vi "Led Comm.vi"() -> ()   [LabVIEW 2019]
uses:
  <vilib>/Rock Robotics/WPI/DriverStation/WPI_DriverStationRobotMode2.ctl
  <vilib>/Rock Robotics/SystemInterfaces/DIO/FPGA_DIOChannel.ctl
  Robot Global Data.vi
panel:
  in  "number":i32
  in  "Time Left":sgl
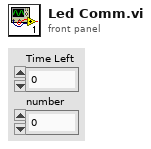
[diagram p1: front panel]
types:
  T1 = typedef "FPGA_DIOChannel.ctl" = enum8{"DIO 0", "DIO 1", "DIO 2", "DIO 3", "DIO 4", "DIO 5", "DIO 6", "DIO 7", "DIO 8", "DIO 9", "DIO MXP 0", "DIO MXP 1", "DIO MXP 2", "DIO MXP 3", "DIO MXP 4", "DIO MXP 5", "DIO MXP 6", "DIO MXP 7", "DIO MXP 8", "DIO MXP 9", "DIO MXP 10", "DIO MXP 11", "DIO MXP 12", "DIO MXP 13", "DIO MXP 14", "DIO MXP 15", "SPI Port CS1", "SPI Port CS2", "SPI Port CS3", "SPI Port MISO", "SPI Port MOSI", "Invalid"}
  T2 = typedef "WPI_DriverStationRobotMode2.ctl" = enum16{"Autonomous Disabled", "Autonomous Enabled", "Teleop Disabled", "Teleop Enabled", "Disconnected", "Finish", "Test Disabled", "Test Enabled", "Emergency Stopped"}
  T3 = typedef "WPI_DigitalOutputDevRef.ctl" = cluster{"DIO Channel":T1, "DevStatus":errorcluster}
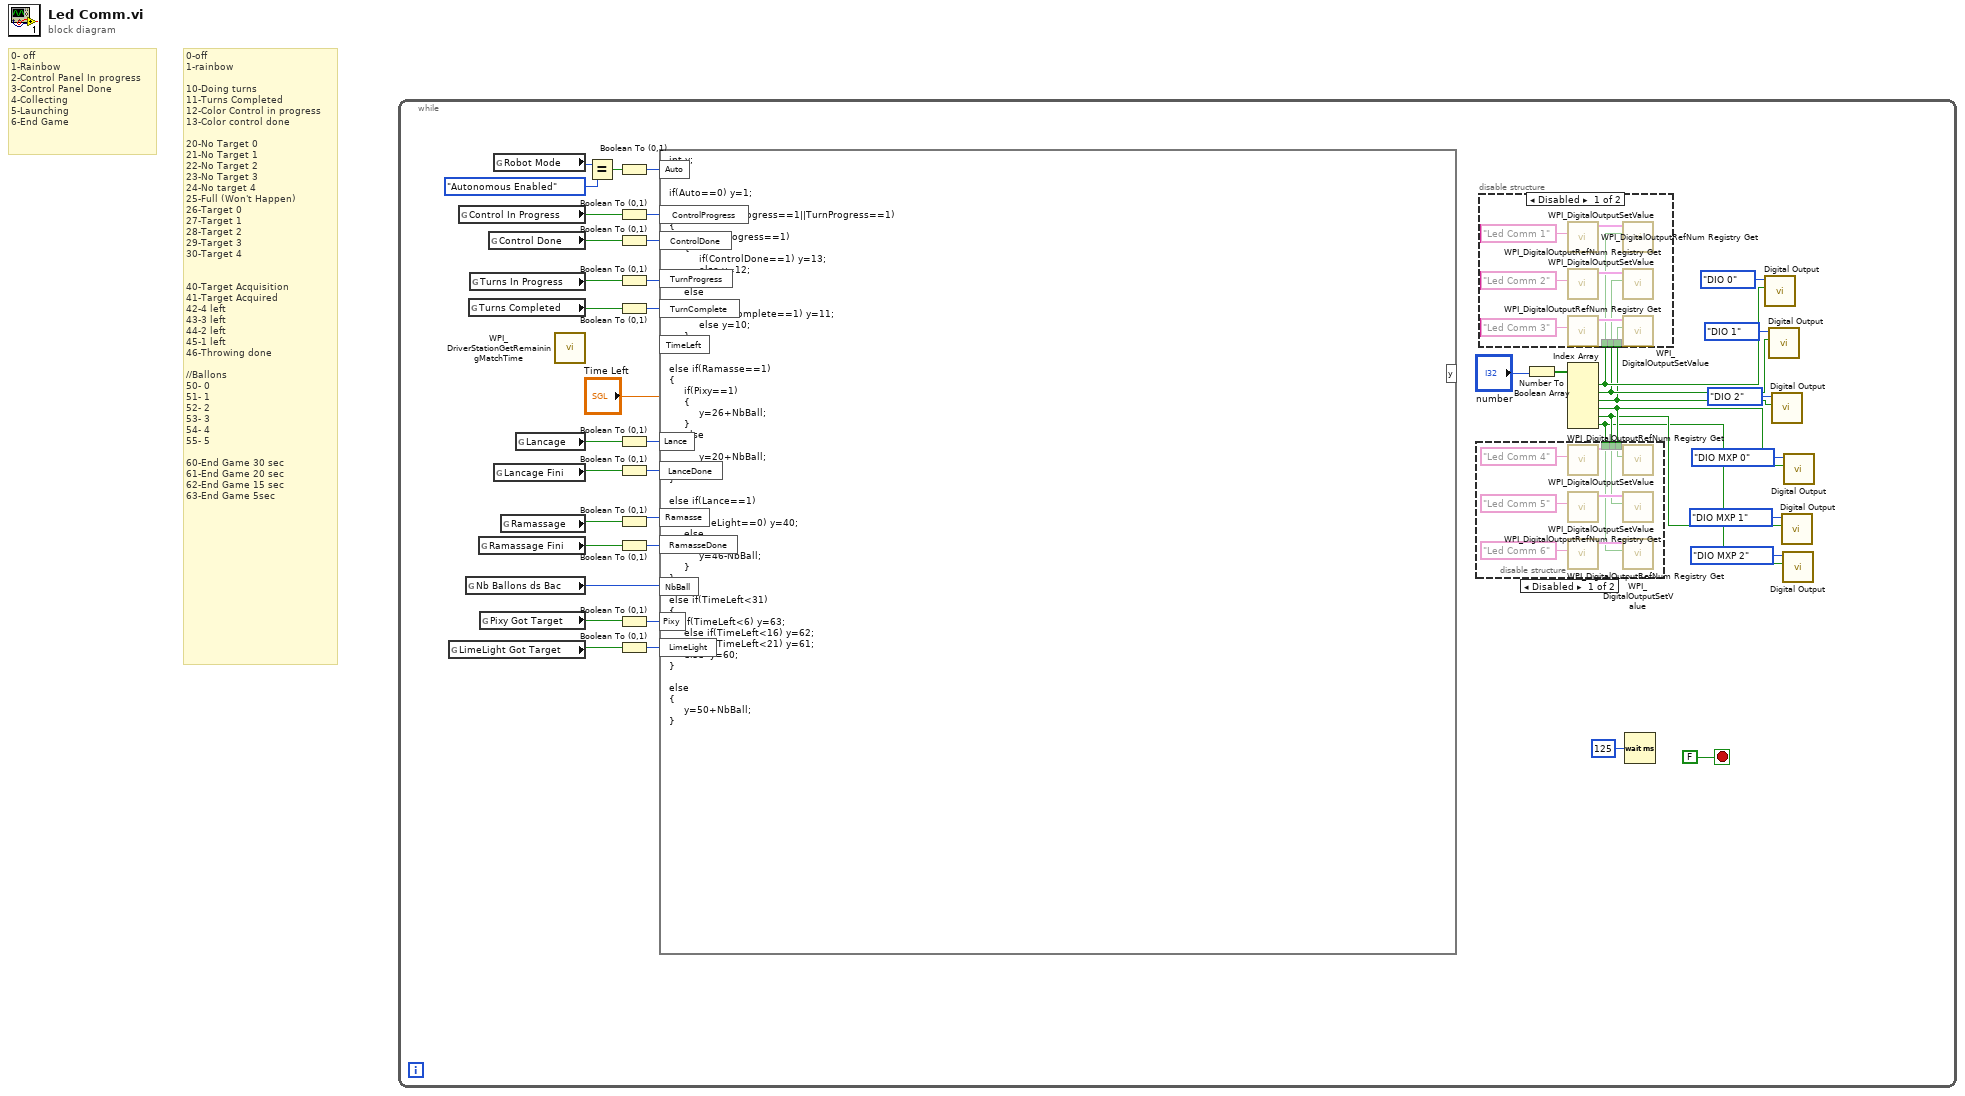
[diagram p0: block diagram]
diagram:
  # "0-off\n1-rainbow\n\n10-Doing turns\n11-Turns Completed\n12-Color Control in progress\n13-Color control done\n\n20-No Target 0\n21-No Target 1\n22-No Target 2\n23-No Target 3\n24-No target 4\n25-Full (Won't Happen)\n26-Target 0\n27-Target 1\n28-Target 2\n29-Target 3\n30-Target 4\n\n\n40-Target Acquisition\n41-Target Acquired\n42-4 left\n43-3 left\n44-2 left\n45-1 left\n46-Throwing done\n\n//Ballons\n50- 0\n51- 1\n52- 2\n53- 3\n54- 4\n55- 5\n\n60-End Game 30 sec\n61-End Game 20 sec\n62-End Game 15 sec\n63-End Game 5sec"
  # "0- off\n1-Rainbow\n2-Control Panel In progress\n3-Control Panel Done\n4-Collecting\n5-Launching\n6-End Game"
  n1 = while {
    stop <- FALSE stop-if-true
    n2 = global read "Robot Global Data.vi" "LimeLight Got Target"() -> (w23:bool)
    n3 = global read "Robot Global Data.vi" "Control In Progress"() -> (w18:bool)
    n4 = global read "Robot Global Data.vi" "Nb Ballons ds Bac"() -> (w24:u8)
    n5 = global read "Robot Global Data.vi" "Turns Completed"() -> (w35:bool)
    n6 = global read "Robot Global Data.vi" "Turns In Progress"() -> (w19:bool)
    n7 = global read "Robot Global Data.vi" "Ramassage Fini"() -> (w34:bool)
    n8 = global read "Robot Global Data.vi" "Pixy Got Target"() -> (w22:bool)
    n9 = global read "Robot Global Data.vi" "Control Done"() -> (w40:bool)
    n10 = global read "Robot Global Data.vi" "Robot Mode"() -> (w38:T2)
    n11 = global read "Robot Global Data.vi" "Lancage Fini"() -> (w39:bool)
    n12 = global read "Robot Global Data.vi" "Ramassage"() -> (w33:bool)
    n13 = global read "Robot Global Data.vi" "Lancage"() -> (w32:bool)
    n14 = call <vilib>:"WPI_DriverStationGetRemainingMatchTime.vi"() -> ()  [unwired: 10 in, 2 out]
    n15 = Equal?(x=w38, y=WPI_DriverStationRobotMode2."Autonomous Enabled") -> (x = y?=w36:bool)
    n16 = Boolean To (0,1)(Boolean=w36) -> (0, 1=w31:i16)
    n17 = Boolean To (0,1)(Boolean=w18) -> (0, 1=w16:i16)
    n18 = Boolean To (0,1)(Boolean=w40) -> (0, 1=w30:i16)
    n19 = Boolean To (0,1)(Boolean=w19) -> (0, 1=w17:i16)
    n20 = Boolean To (0,1)(Boolean=w35) -> (0, 1=w29:i16)
    n21 = Boolean To (0,1)(Boolean=w32) -> (0, 1=w28:i16)
    n22 = Boolean To (0,1)(Boolean=w39) -> (0, 1=w27:i16)
    n23 = Boolean To (0,1)(Boolean=w33) -> (0, 1=w26:i16)
    n24 = Boolean To (0,1)(Boolean=w34) -> (0, 1=w25:i16)
    n25 = Boolean To (0,1)(Boolean=w22) -> (0, 1=w21:i16)
    n26 = Boolean To (0,1)(Boolean=w23) -> (0, 1=w20:i16)
    n27 = formula code="int y;\ny=0;\n\nif(Auto==0) y=1;\n\nelse if(ControlProgress==1||TurnProgress==1)\n{\n   if(ControlProgress==1)\n     {\n          if(ControlDone==1) y=13;\n          else y=12;\n     }\n     else\n     {\n          if(TurnComplete==1) y=11;\n          else y=10;\n     }\n}\n\nelse if(Ramasse==1)\n{\n     if(Pixy==1)\n     {\n          y=26+NbBall;\n     }\n     else\n     {\n          y=20+NbBall;\n     }\n}\n\nelse if(Lance==1)\n{\n     if(LimeLight==0) y=40;\n     else\n     {\n          y=46-NbBall;\n     }\n}\n\nelse if(TimeLeft<31)\n{\n     if(TimeLeft<6) y=63;\n     else if(TimeLeft<16) y=62;\n     else if(TimeLeft<21) y=61;\n     else  y=60;\n}\n\nelse\n{\n     y=50+NbBall;\n}"("ControlDone"=w30, "TurnComplete"=w29, "TimeLeft"="Time Left", "Auto"=w31, "Lance"=w28, "LanceDone"=w27, "Ramasse"=w26, "RamasseDone"=w25, "NbBall"=w24, "Pixy"=w21, "LimeLight"=w20, "ControlProgress"=w16, "TurnProgress"=w17) -> ()  [unwired: 1 out]
    n28 = Number To Boolean Array(number="number") -> (Boolean array=w41:bool[])
    n29 = Index Array(array=w41) -> (element #1=w12:bool, element #2=w11:bool, element #3=w10:bool, element #4=w9:bool, element #5=w8:bool, element #6=w7:bool)  [unwired: 6 in]
    n30 = disable-structure shown="Disabled" {
      disable-tunnel: w9 -> [w45 _]
      disable-tunnel: w8 -> [w44 _]
      disable-tunnel: w7 -> [w43 _]
      frame Disabled {
        n31 = call <vilib>:"WPI_DigitalOutputRefNum Registry Get.vi"("refnum name"="Led Comm 4") -> ("DigitalOutputDevRef"=w48:T3)  [unwired: 9 in, 1 out]
        n32 = call <vilib>:"WPI_DigitalOutputRefNum Registry Get.vi"("refnum name"="Led Comm 5") -> ("DigitalOutputDevRef"=w47:T3)  [unwired: 9 in, 1 out]
        n33 = call <vilib>:"WPI_DigitalOutputRefNum Registry Get.vi"("refnum name"="Led Comm 6") -> ("DigitalOutputDevRef"=w46:T3)  [unwired: 9 in, 1 out]
        n34 = call <vilib>:"WPI_DigitalOutputSetValue.vi"("Value"=w45, "DigitalOutputDevRef"=w48) -> ()  [unwired: 8 in, 2 out]
        n35 = call <vilib>:"WPI_DigitalOutputSetValue.vi"("Value"=w44, "DigitalOutputDevRef"=w47) -> ()  [unwired: 8 in, 2 out]
        n36 = call <vilib>:"WPI_DigitalOutputSetValue.vi"("Value"=w43, "DigitalOutputDevRef"=w46) -> ()  [unwired: 8 in, 2 out]
      }
      frame Enabled {
      }
    }
    n37 = disable-structure shown="Disabled" {
      disable-tunnel: w12 -> [w54 _]
      disable-tunnel: w11 -> [w53 _]
      disable-tunnel: w10 -> [w52 _]
      frame Disabled {
        n38 = call <vilib>:"WPI_DigitalOutputRefNum Registry Get.vi"("refnum name"="Led Comm 1") -> ("DigitalOutputDevRef"=w57:T3)  [unwired: 9 in, 1 out]
        n39 = call <vilib>:"WPI_DigitalOutputRefNum Registry Get.vi"("refnum name"="Led Comm 2") -> ("DigitalOutputDevRef"=w56:T3)  [unwired: 9 in, 1 out]
        n40 = call <vilib>:"WPI_DigitalOutputRefNum Registry Get.vi"("refnum name"="Led Comm 3") -> ("DigitalOutputDevRef"=w55:T3)  [unwired: 9 in, 1 out]
        n41 = call <vilib>:"WPI_DigitalOutputSetValue.vi"("Value"=w54, "DigitalOutputDevRef"=w57) -> ()  [unwired: 8 in, 2 out]
        n42 = call <vilib>:"WPI_DigitalOutputSetValue.vi"("Value"=w53, "DigitalOutputDevRef"=w56) -> ()  [unwired: 8 in, 2 out]
        n43 = call <vilib>:"WPI_DigitalOutputSetValue.vi"("Value"=w52, "DigitalOutputDevRef"=w55) -> ()  [unwired: 8 in, 2 out]
      }
      frame Enabled {
      }
    }
    n44 = Wait (ms)(milliseconds to wait=u32 125) -> ()  [unwired: 1 out]
    n45 = call <vilib>:"Digital Output.vi"("DO State"=w12, "DIO Channel"=FPGA_DIOChannel."DIO 0") -> ()  [unwired: 10 in]
    n46 = call <vilib>:"Digital Output.vi"("DO State"=w11, "DIO Channel"=FPGA_DIOChannel."DIO 1") -> ()  [unwired: 10 in]
    n47 = call <vilib>:"Digital Output.vi"("DO State"=w10, "DIO Channel"=FPGA_DIOChannel."DIO 2") -> ()  [unwired: 10 in]
    n48 = call <vilib>:"Digital Output.vi"("DO State"=w8, "DIO Channel"=FPGA_DIOChannel."DIO MXP 1") -> ()  [unwired: 10 in]
    n49 = call <vilib>:"Digital Output.vi"("DO State"=w7, "DIO Channel"=FPGA_DIOChannel."DIO MXP 2") -> ()  [unwired: 10 in]
    n50 = call <vilib>:"Digital Output.vi"("DO State"=w9, "DIO Channel"=FPGA_DIOChannel."DIO MXP 0") -> ()  [unwired: 10 in]
  }
